vi "Check Trigger Conditions.vi"(7 "Force Trigger?":bool, 8 "error in (no error)":errorcluster, 9 "Waveform Data":waveform(sgl)[](array[waveform]), 10 "Acquisition and Logging Configuration":T1={"Data Rate"=1, "Samples per Read"=0, "Number of Reads to Save"=0, "Data File Name"="", "TDMS Properties"=[], "Number of Channels"=4, "Channel Scale Array"=[0.0, 0.0, 0.0, 0.0, 1.0, 1.0, 1.0, 1.0, 1.0, 1.0, 1.0, 1.0, 1.0, 1.0, 1.0, 1.0, 1.0, 1.0, 1.0, 1.0, 1.0, 1.0, 1.0, 1.0], "Channel Names"=[], "Trigger - RMS Value"=0.0, "Trigger - Channel"=0, "Trigger - Time (Minute)"=0} {"Data Rate" items=["51.200 kS/s (NI 9234)"=1, "25.600 kS/s (NI 9234)"=2, "17.067 kS/s (NI 9234)"=3, "12.800 kS/s (NI 9234)"=4, "10.240 kS/s (NI 9234)"=5, "8.533 kS/s (NI 9234)"=6, "7.314 kS/s (NI 9234)"=7, "6.400 kS/s (NI 9234)"=8, "5.689 kS/s (NI 9234)"=9, "5.120 kS/s (NI 9234)"=10, "4.654 kS/s (NI 9234)"=11, "4.267 kS/s (NI 9234)"=12, "3.938 kS/s (NI 9234)"=13, "3.657 kS/s (NI 9234)"=14, "3.413 kS/s (NI 9234)"=15, "3.200 kS/s (NI 9234)"=16, "3.012 kS/s (NI 9234)"=17, "2.845 kS/s (NI 9234)"=18, "2.695 kS/s (NI 9234)"=19, "2.560 kS/s (NI 9234)"=20, "2.438 kS/s (NI 9234)"=21, "2.328 kS/s (NI 9234)"=22, "2.226 kS/s (NI 9234)"=23, "2.133 kS/s (NI 9234)"=24, "2.048 kS/s (NI 9234)"=25, "1.969 kS/s (NI 9234)"=26, "1.896 kS/s (NI 9234)"=27, "1.829 kS/s (NI 9234)"=28, "1.765 kS/s (NI 9234)"=29, "1.707 kS/s (NI 9234)"=30, "1.652 kS/s (NI 9234)"=31]}) -> (0 "error out":errorcluster, 3 "Trigger Condition Met?":bool)   [LabVIEW 2015]
uses:
  controls/Acquisition and Logging Configuration.ctl
  <vilib>/LabVIEW Targets/FPGA/cRIO/shared/nicrio_ModuleControls/nicrio_cRIO-9234_DataRatesRing2.ctl
  controls/TDMS Properties.ctl
  <vilib>/Analysis/5stat.llb/RMS (DBL).vi
  <vilib>/Analysis/NI_AALPro.lvlib
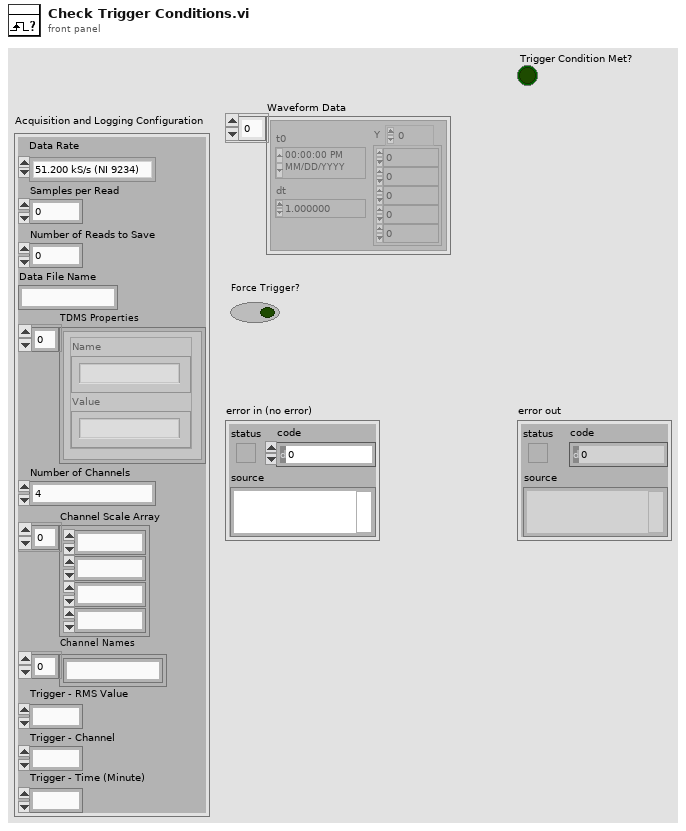
[diagram p1: front panel]
types:
  T1 = typedef "Acquisition and Logging Configuration.ctl" = cluster{"Data Rate":T2, "Samples per Read":i32, "Number of Reads to Save":i32, "Data File Name":string, "TDMS Properties":T3[], "Number of Channels":i32, "Channel Scale Array":fxp<+,24,12>[], "Channel Names":string[], "Trigger - RMS Value":dbl, "Trigger - Channel":i32, "Trigger - Time (Minute)":i32}
  T2 = typedef "nicrio_cRIO-9234_DataRatesRing2.ctl" = u8
  T3 = typedef "TDMS Properties.ctl" = cluster{"Name":string, "Value":string}
  T4 = typedef "LVDateTimeRec.ctl" = cluster{"fractional second":dbl, "second":i32, "minute":i32, "hour":i32, "day of month":i32, "month":i32, "year":i32, "day of week":i32, "day of year":i32, "DST":i32}
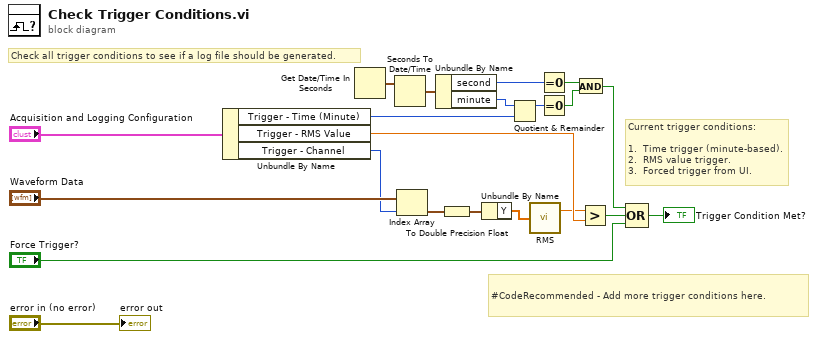
[diagram p0: block diagram]
diagram:
  # "Check all trigger conditions to see if a log file should be generated."
  # "Current trigger conditions:\n\n1.  Time trigger (minute-based).\n2.  RMS value trigger.\n3.  Forced trigger from UI."
  # "#CodeRecommended - Add more trigger conditions here."
  n1 = Unbundle By Name("Acquisition and Logging Configuration") -> ("Trigger - Time (Minute)"=w5:i32, "Trigger - RMS Value"=w18:dbl, "Trigger - Channel"=w17:i32)
  n2 = Get Date/Time In Seconds() -> (seconds since 1Jan1904=w7:timestamp)
  n3 = Seconds To Date/Time(time stamp (now)=w7) -> (date time rec=w13:T4)  [unwired: 1 out]
  n4 = Index Array(array="Waveform Data", index=w17) -> (element=w16:waveform(sgl))
  n5 = Unbundle By Name(w13) -> ("second"=w12:i32, "minute"=w11:i32)
  n6 = To Double Precision Float(number=w16) -> (double precision float=w15:waveform(dbl))
  n7 = Unbundle By Name(w15) -> ("Y"=w2:dbl[])
  n8 = Quotient & Remainder(x=w11, y=w5) -> (x-y*floor(x/y)=w10:i32)  [unwired: 1 out]
  n9 = call-poly <vilib>:"RMS.vi"("X"=w2) -> ("rms value"=w1:dbl)  [unwired: 1 out]
  n10 = Equal To 0?(x=w12) -> (x = 0?=w9:bool)
  n11 = Equal To 0?(x=w10) -> (x = 0?=w8:bool)
  n12 = And(x=w9, y=w8) -> (x .and. y?=w4:bool)
  n13 = Greater?(x=w1, y=w18) -> (0:w14:bool)
  n14 = Compound Arithmetic op=OR(w4, w14, "Force Trigger?") -> (→"Trigger Condition Met?":bool)
  "error out" <- "error in (no error)"
